vi "Apply Signal Names.vi"(8 "error in":errorcluster, 11 "2575 in":refnum<class "2575.lvclass">) -> (0 "error out":errorcluster, 3 "2575 out":refnum<class "2575.lvclass">)   [LabVIEW 2019]
uses:
  Library/2575.lvclass
  C:/Users/Public/Documents/Development/builds/Instruments/SwitchMatrix.lvlibp/Library/SwitchMatrix.lvclass
  C:/Users/Public/Documents/Development/builds/Tools/Config.lvlibp/Config.lvclass
  builds/Instruments/SwitchMatrix.lvlibp/Accessors/Read Relay Name.vi
  builds/Tools/Config.lvlibp/Accessors/Read Device Signals.vi
  builds/Instruments/SwitchMatrix.lvlibp/Library/SwitchMatrix.lvclass
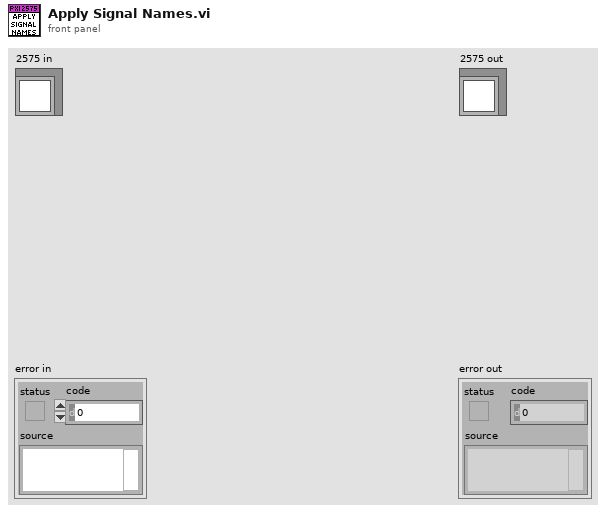
[diagram p1: front panel]
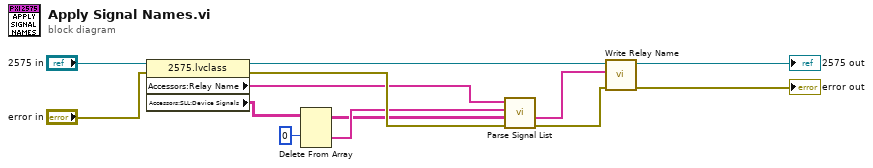
[diagram p0: block diagram]
diagram:
  n1 = property class="2575.lvclass"(reference="2575 in", error in="error in") -> (reference out=w8:refnum<class "2575.lvclass">, error out=w9:errorcluster, "Accessors:Relay Name"=w5:string[], "Accessors:SLL:Device Signals"=w4:string[][])
  n2 = Delete From Array(array=w4, index (row)=0) -> (deleted portion=w2:string[], array with subset deleted=w1:string[][])  [unwired: 2 in]
  n3 = call "Parse Signal List.vi"("error in (no error)"=w9, "Signal List"=w1, "Headers"=w2, "Relay Names"=w5) -> ("error out"=w6:errorcluster, "Names"=w7:string[])  [unwired: 6 in]
  n4 = call "Write Relay Name.vi"("error in (no error)"=w6, "Relay Name"=w7, "SwitchMatrix in"=w8) -> ("error out"=→"error out":errorcluster, "SwitchMatrix out"=→"2575 out":refnum<class "2575.lvclass">)  [unwired: 7 in]
